vi "Main.vi"() -> ()   [LabVIEW 2020]
panel:
  out "error out":errorcluster
  in  "Teach 2-1":T1
  in  "Teach 1-1":T2
  in  "Help":bool
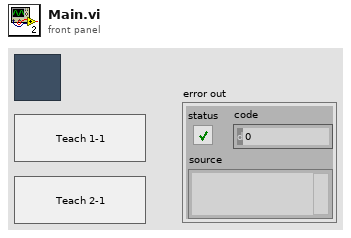
[diagram p1: front panel]
types:
  T1 = typedef "Teach 2-1.ctl" = bool
  T2 = typedef "Teach 1-1.ctl" = bool
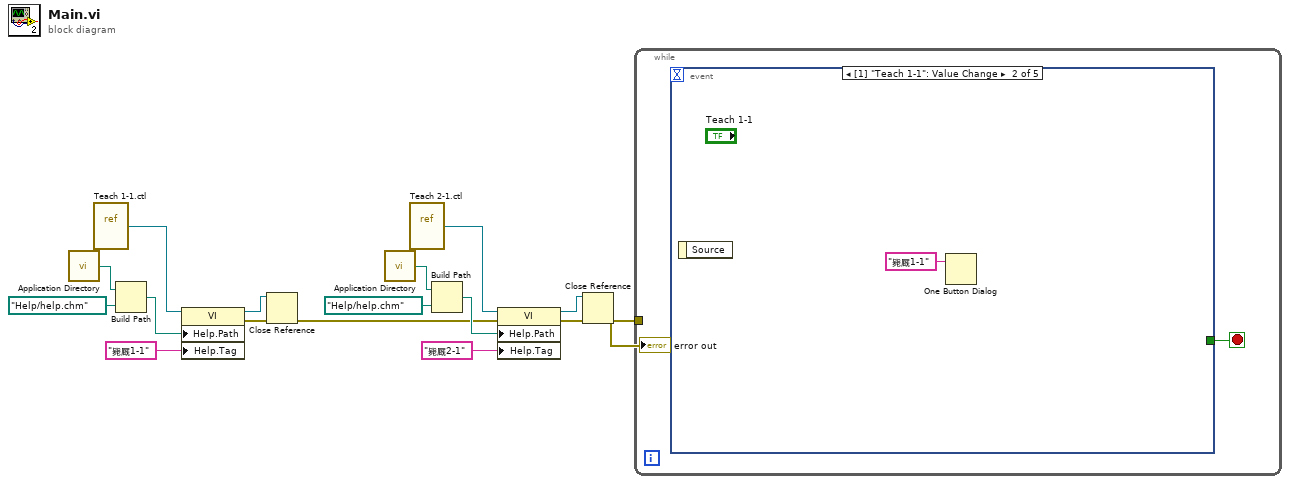
[diagram p0: block diagram]
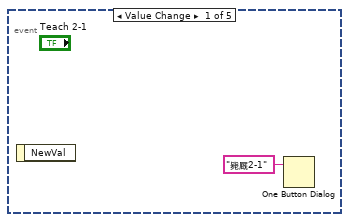
[diagram p2: hidden frame]
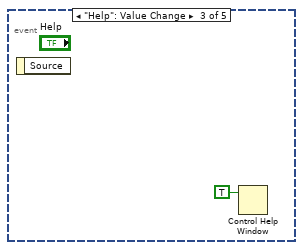
[diagram p3: hidden frame]
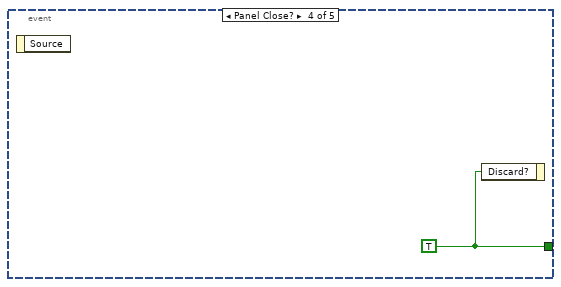
[diagram p4: hidden frame]
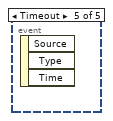
[diagram p5: hidden frame]
diagram:
  n1 = call <vilib>:"Application Directory.vi"() -> ("Application Directory"=w15:path)
  n2 = vi-ref "Teach 1-1.ctl"() -> (w16:refnum<vi>)
  n3 = Build Path(base path=w15, name or relative path=path "Help/help.chm") -> (appended path=w13:path)
  n4 = property class="VI"(reference=w16, "Help.Path"=w13, "Help.Tag"="毙厩1-1" ("Help:Document Tag")) -> (reference out=w11:refnum<vi>, error out=w12:errorcluster)  [unwired: 1 in]
  n5 = Close Reference(reference=w11, error in (no error)=w12) -> (error out=w4:errorcluster)
  n6 = call <vilib>:"Application Directory.vi"() -> ("Application Directory"=w6:path)
  n7 = vi-ref "Teach 2-1.ctl"() -> (w5:refnum<vi>)
  n8 = Build Path(base path=w6, name or relative path=path "Help/help.chm") -> (appended path=w8:path)
  n9 = property class="VI"(reference=w5, error in=w4, "Help.Path"=w8, "Help.Tag"="毙厩2-1" ("Help:Document Tag")) -> (reference out=w10:refnum<vi>, error out=w9:errorcluster)
  n10 = Close Reference(reference=w10, error in (no error)=w9) -> (error out=w3:errorcluster)
  "error out" <- w3
  n11 = while {
    tunnel: w3 -> [_]
    stop <- w17 stop-if-true
    n12 = event shown="[1] \"Teach 1-1\": Value Change" {
      selector: _ -> [_ _ _ _ _]
      dyn-events: _ -> [_ _ _ _ _]
      timeout: _ -> [_ _ _ _ _]
      tunnel: [_ _ _ w21 _] -> w17
      event Value Change {
        n13 = event-data() -> ()  [unwired: 1 in, 1 out]
        n14 = One Button Dialog(message="毙厩2-1") -> ()  [unwired: 1 in, 1 out]
      }
      event Value Change {
        n15 = event-data() -> ()  [unwired: 1 in, 1 out]
        n16 = One Button Dialog(message="毙厩1-1") -> ()  [unwired: 1 in, 1 out]
      }
      event "Help": Value Change {
        n17 = event-data() -> ()  [unwired: 1 in, 1 out]
        n18 = Control Help Window(1:TRUE ("Show")) -> ()  [unwired: 1 in]
      }
      event Panel Close? {
        w21 = TRUE
        n19 = event-data() -> ()  [unwired: 1 in, 1 out]
        n20 = event-data("Discard?"=w21) -> ()  [unwired: 1 in, 1 out]
      }
      event Timeout {
        n21 = event-data() -> ()  [unwired: 1 in, 3 out]
      }
    }
  }
